vi "Disconnect.vi"(8 "ErrorArray":errorcluster[](array[cluster])) -> (0 "ErrorArray":errorcluster[](array[cluster]))   [LabVIEW 2014, in "Comms.lvlib"]
uses:
  Comms.lvlib
  <userlib>/NIST/Socket Class/Classes/Socket.TCP/Socket.TCP.lvclass
  <userlib>/NIST/NISTErrorLib/NISTErrorLib.lvlib
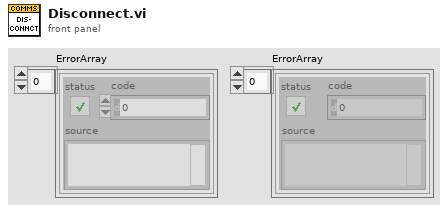
[diagram p1: front panel]
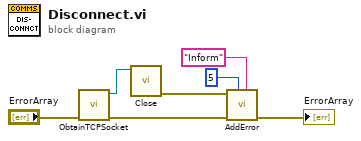
[diagram p0: block diagram]
diagram:
  n1 = call "ObtainTCPSocket.vi"("ErrorArray"="ErrorArray") -> ("ErrorArray"=w6:errorcluster[], "SocketRef"=w4:refnum<class "Socket.TCP.lvclass">)  [unwired: 9 in]
  n2 = call-dynamic "Close.vi"("Socket.TCP in"=w4) -> ("error out"=w3:errorcluster)  [unwired: 9 in, 1 out]
  n3 = call <userlib>:"AddError.vi"("Severity"="Inform", "Priority"=u8 5, "ErrorArray"=w6, "error in (no error)"=w3) -> ("ErrorArray"=→"ErrorArray":errorcluster[])  [unwired: 6 in, 1 out]
